vi "CBSControlling.vi"() -> ()   [LabVIEW 2017]
uses:
  classes/DataHandlerMYiTOPS.lvclass
panel:
  in  "Monitoring":T1 {"Meter" scale=0.0..20.0}
  out "appended array":string[](array[string])
  out "element":string
  out "Control-Matrix-Overview 2":i32(listbox)=-1
  in  "Controlling":T2
  in  "Cyber-physical Objects":i32(listbox)
  in  "Stop":bool
  out "Control-Matrix-Overview":i32(listbox)=-1
  # "Hard Key:"
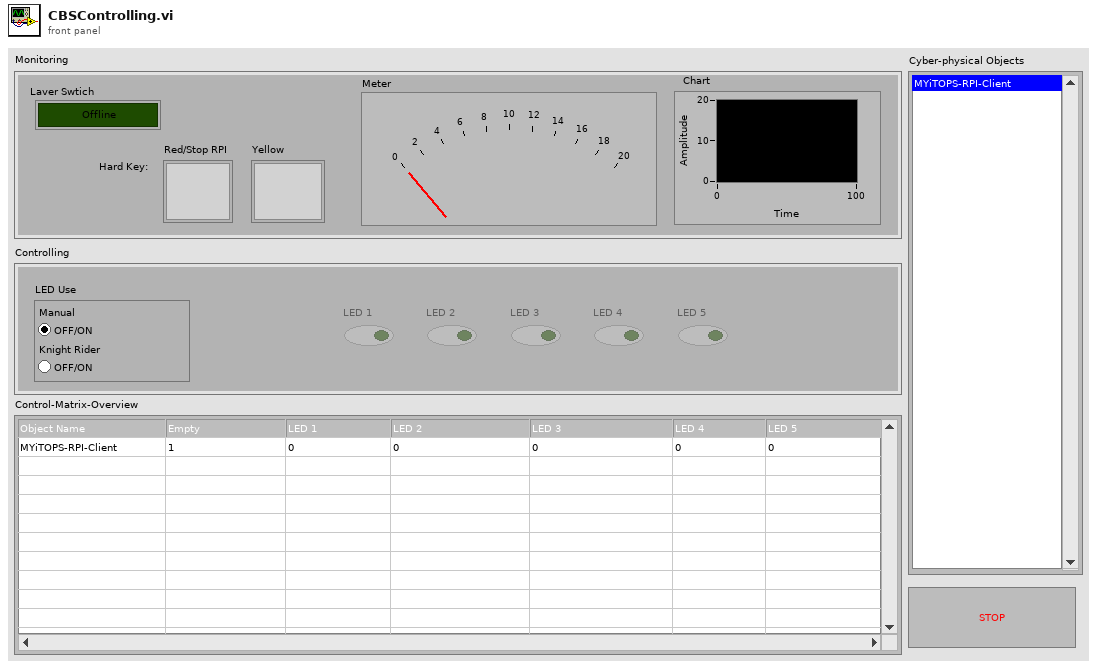
[diagram p1: front panel]
types:
  T1 = cluster{"Meter":i8, "Chart":dbl, "Yellow":bool, "Red/Stop RPI":bool, "Laver Swtich":bool}
  T2 = cluster{"LED 1":bool, "LED 5":bool, "LED 2":bool, "LED 3":bool, "LED 4":bool, "LED Use":enum32{"Manual", "Knight Rider"}}
  T3 = enum8{"Enabled", "Disabled", "Disabled and Grayed Out"}
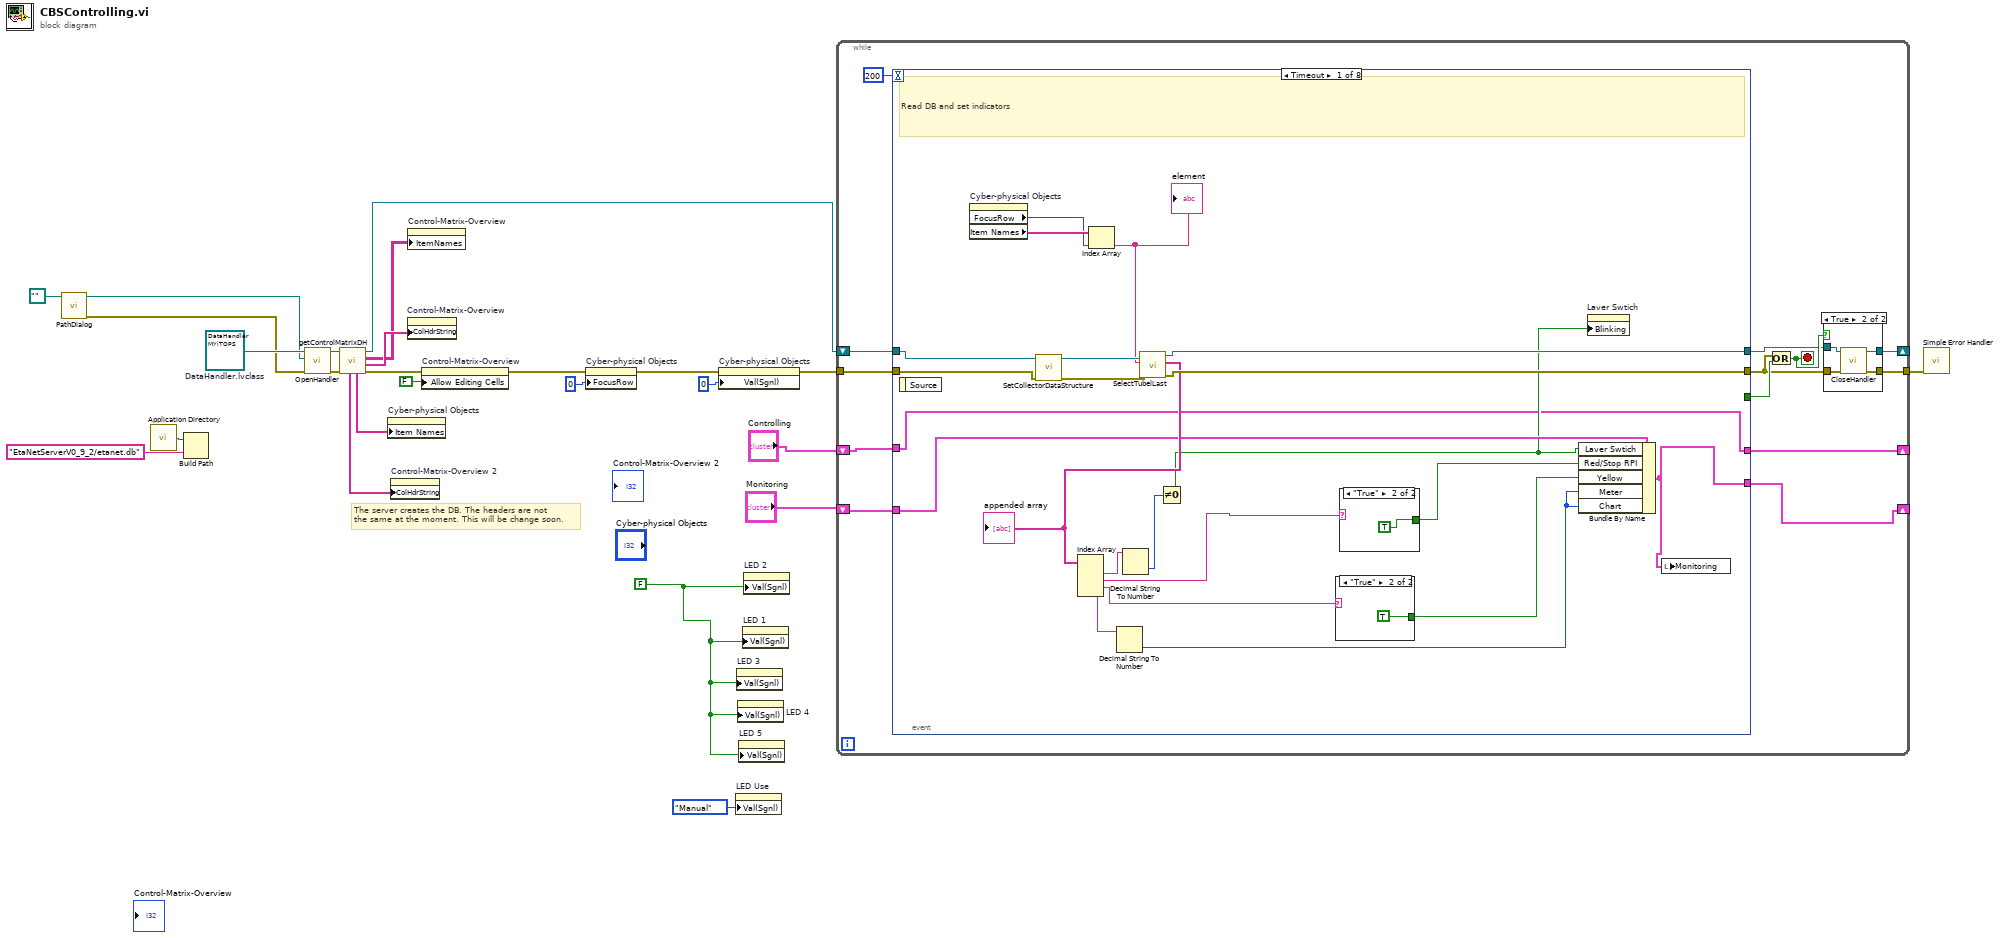
[diagram p0: block diagram]
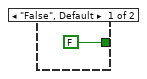
[diagram p3: hidden frame]
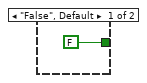
[diagram p4: hidden frame]
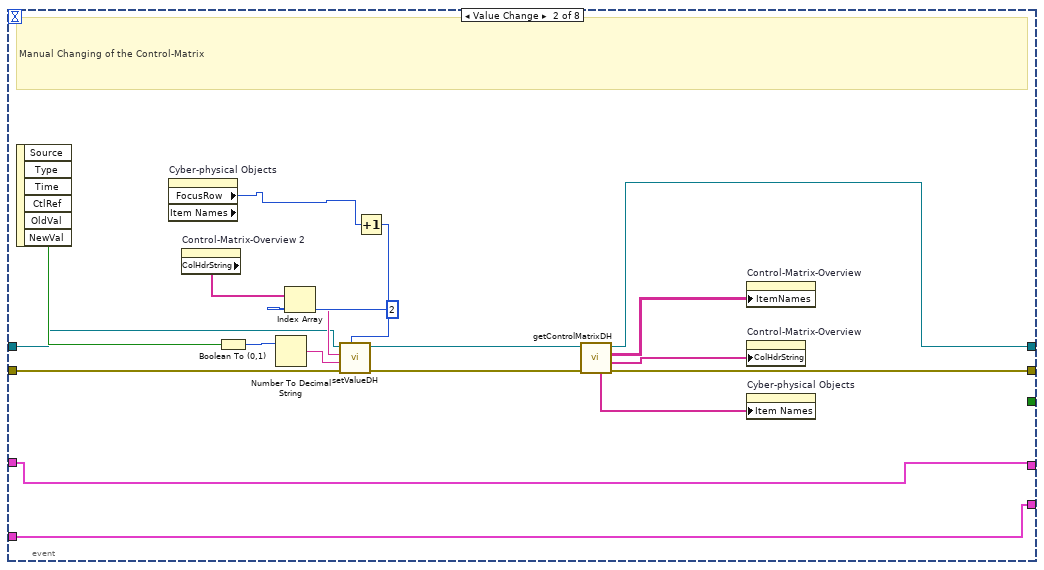
[diagram p5: hidden frame]
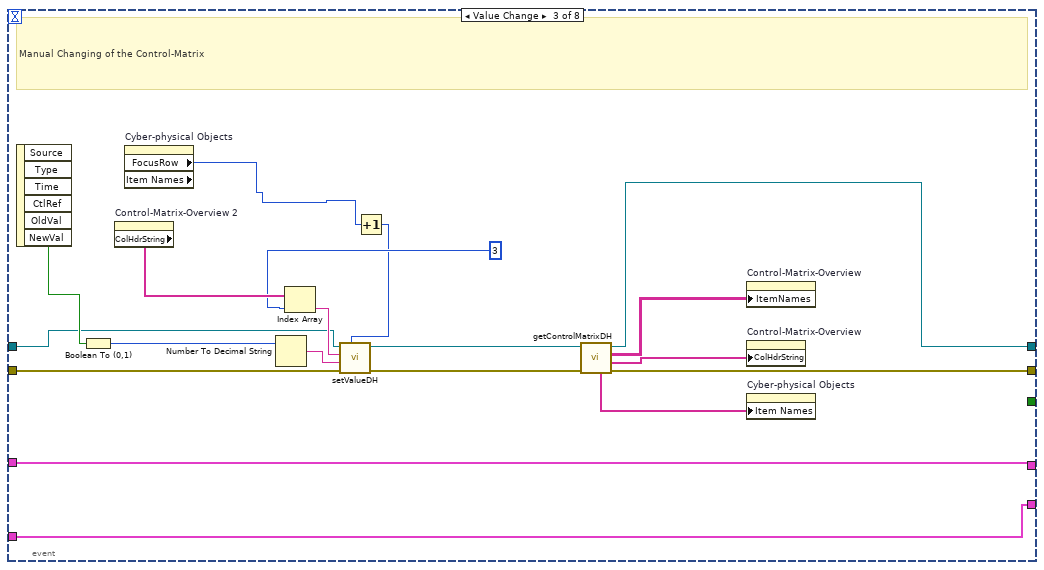
[diagram p6: hidden frame]
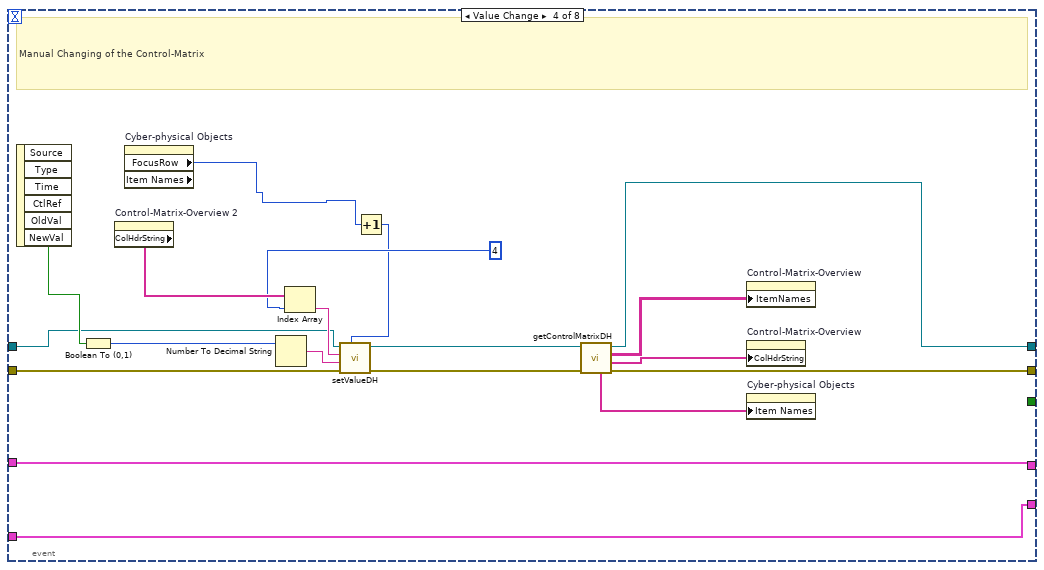
[diagram p7: hidden frame]
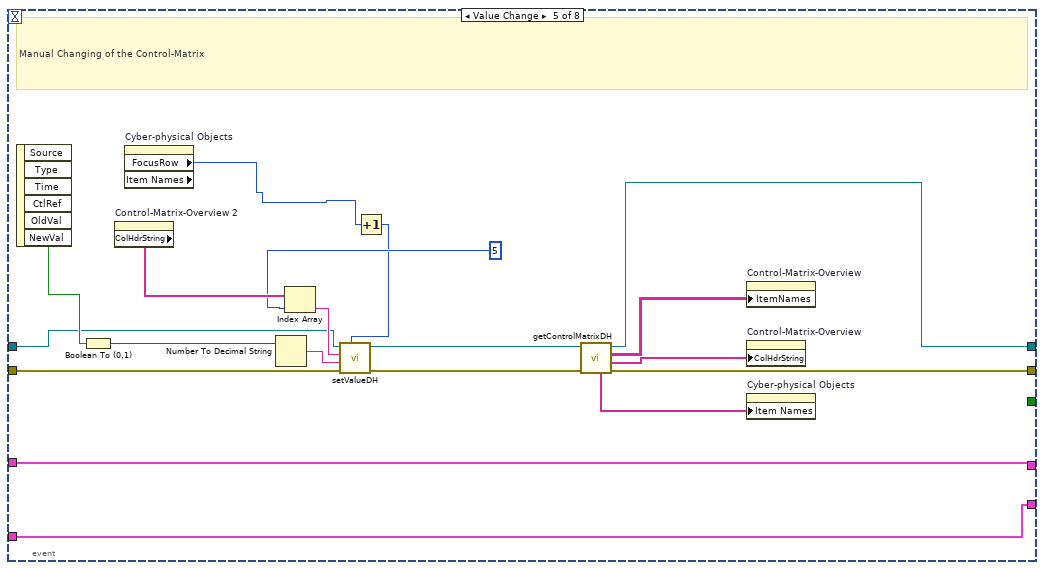
[diagram p8: hidden frame]
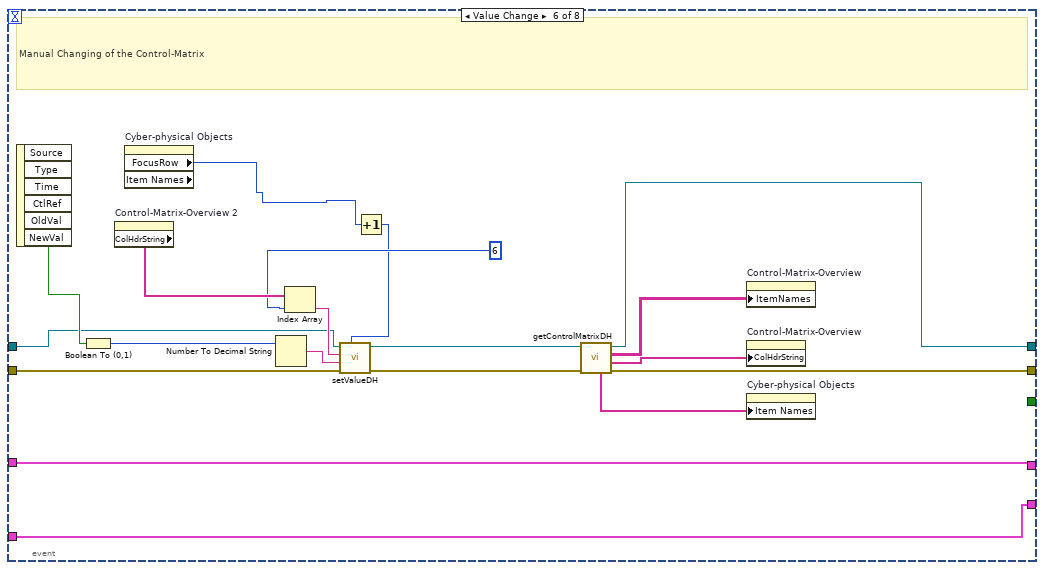
[diagram p9: hidden frame]
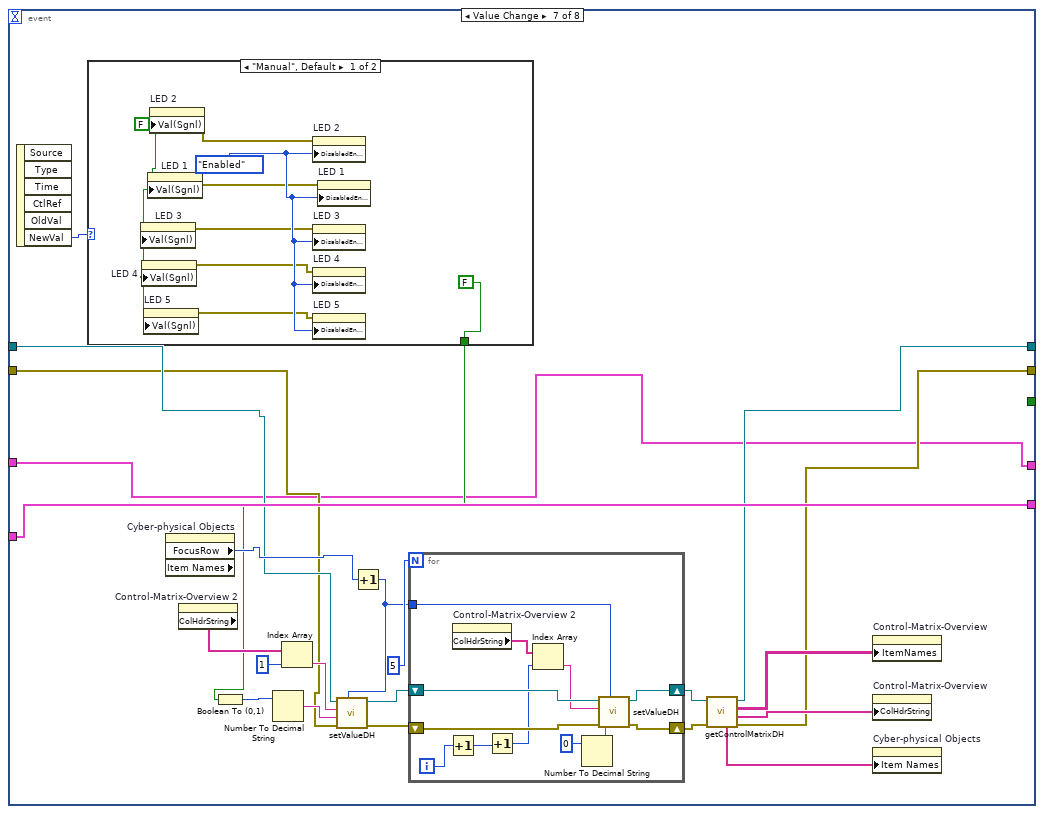
[diagram p10: hidden frame]
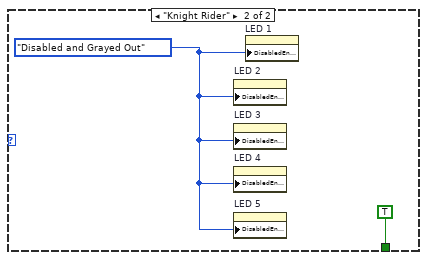
[diagram p11: hidden frame]
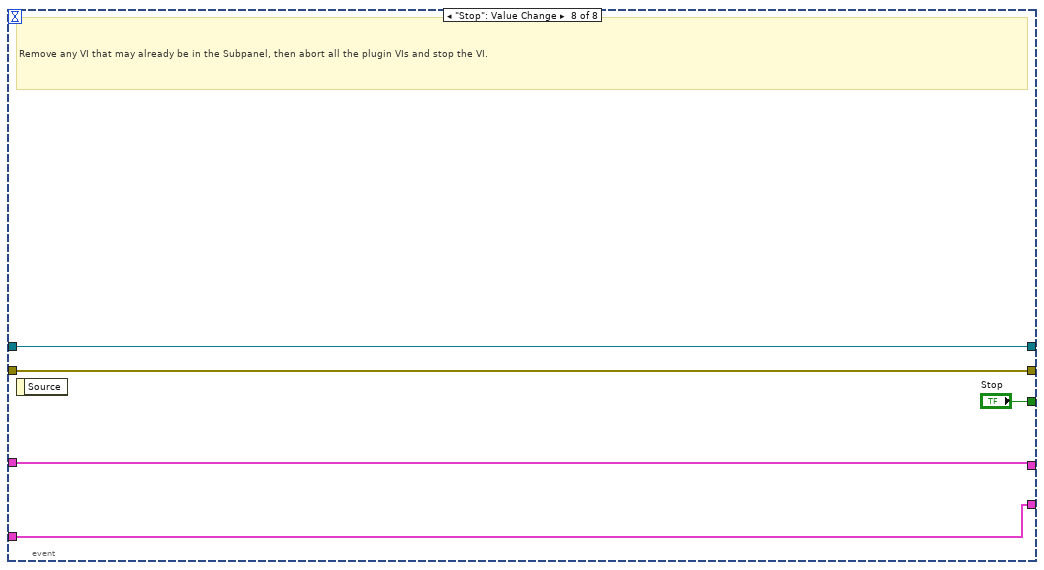
[diagram p12: hidden frame]
diagram:
  w4 = FALSE ("Value")
  w20 = refnum<class "DataHandlerMYiTOPS.lvclass"> refnum  # DataHandler.lvclass
  # "The server creates the DB. The headers are not \nthe same at the moment. This will be change soon."
  n1 = call "PathDialog.vi"("Path to Data Base in"=path "" ("Path to Data Base")) -> ("error out"=w2:errorcluster, "Path to Data Base out"=w6:path)  [unwired: 9 in]
  n2 = call <vilib>:"Application Directory.vi"() -> ("Application Directory"=w21:path)
  n3 = Build Path(base path=w21, name or relative path="EtaNetServerV0_9_2/etanet.db" ("Name oder relativer Pfad")) -> ()  [unwired: 1 out]
  n4 = call-dynamic "OpenHandler.vi"("error in (no error)"=w2, "path to db monitoring"=w6, "DataHandling in"=w20) -> ("error out"=w18:errorcluster, "DataHandling out"=w17:refnum<class "DataHandlerMYiTOPS.lvclass">)  [unwired: 7 in]
  n5 = call-dynamic "getControlMatrixDH.vi"("error in (no error)"=w18, "DataHandler in"=w17) -> ("error out"=w15:errorcluster, "List of ColHads"=w14:string[], "Array"=w9:string[][], "DataHandler out"=w10:refnum<class "DataHandlerMYiTOPS.lvclass">, "Field Elements"=w16:string[], "List of ColHads 2"=w8:string[])  [unwired: 4 in]
  n6 = property on="Cyber-physical Objects" class="LstBox (strict)"("Item Names"=w16) -> ()  [unwired: 2 in, 2 out]
  n7 = property on="Control-Matrix-Overview 2" class="MCListbox (strict)"("ColHdrString"=w8) -> ()  [unwired: 2 in, 2 out]
  n8 = property on="Control-Matrix-Overview" class="MCListbox (strict)"("ColHdrString"=w14) -> ()  [unwired: 2 in, 2 out]
  n9 = property on="Control-Matrix-Overview" class="MCListbox (strict)"("ItemNames"=w9) -> ()  [unwired: 2 in, 2 out]
  n10 = property on="Control-Matrix-Overview" class="MCListbox (strict)"(error in=w15, "Allow Editing Cells"=FALSE) -> (error out=w11:errorcluster)  [unwired: 1 in, 1 out]
  n11 = property on="Cyber-physical Objects" class="LstBox (strict)"(error in=w11, "FocusRow"=0 ("Focus Row")) -> (error out=w12:errorcluster)  [unwired: 1 in, 1 out]
  n12 = property on="Cyber-physical Objects" class="ListBox (strict)"(error in=w12, "Val(Sgnl)"=u16 0 ("Value (Signaling)")) -> (error out=w25:errorcluster)  [unwired: 1 in, 1 out]
  n13 = property on="LED Use" class="RadioBtnsControl (strict)"("Val(Sgnl)"=enum32{"Manual", "Knight Rider"}."Manual" ("Value (Signaling)")) -> ()  [unwired: 2 in, 2 out]
  n14 = property on="LED 3" class="Bool (strict)"("Val(Sgnl)"=w4) -> ()  [unwired: 2 in, 2 out]
  n15 = property on="LED 4" class="Bool (strict)"("Val(Sgnl)"=w4) -> ()  [unwired: 2 in, 2 out]
  n16 = property on="LED 5" class="Bool (strict)"("Val(Sgnl)"=w4) -> ()  [unwired: 2 in, 2 out]
  n17 = property on="LED 1" class="Bool (strict)"("Val(Sgnl)"=w4) -> ()  [unwired: 2 in, 2 out]
  n18 = property on="LED 2" class="Bool (strict)"("Val(Sgnl)"=w4) -> ()  [unwired: 2 in, 2 out]
  n19 = while {
    tunnel: w25 -> [w37]
    tunnel: [w32] -> w23
    shift-right: [w30] -> _
    shift-left: w10 -> [w35]
    shift-right: [w26] -> _
    shift-left: "Controlling" -> [w29]
    shift-right: [w27] -> _
    shift-left: "Monitoring" -> [w28]
    stop <- w34 stop-if-true
    n20 = event shown="[0] Timeout" {
      selector: _ -> [_ _ _ _ _ _ _ _]
      dyn-events: _ -> [_ _ _ _ _ _ _ _]
      timeout: 200 -> [_ _ _ _ _ _ _ _]
      tunnel: [_ _ _ _ _ _ _ "Stop"] -> w38
      tunnel: [w59 w87 w104 w123 w142 w161 w173 w213] -> w33
      tunnel: w37 -> [w61 w89 w108 w127 w146 w165 w174 w213]
      tunnel: w35 -> [w64 w78 w95 w114 w133 w152 w176 w214]
      tunnel: [w62 w79 w96 w115 w134 w153 w175 w214] -> w31
      tunnel: w29 -> [w45 w75 w91 w110 w129 w148 w166 w212]
      tunnel: [w45 w75 w91 w110 w129 w148 w166 w212] -> w26
      tunnel: w28 -> [w49 w74 w90 w109 w128 w147 w187 w211]
      tunnel: [w48 w74 w90 w109 w128 w147 w187 w211] -> w27
      event Timeout {
        # "Read DB and set indicators"
        n21 = event-data() -> ()  [unwired: 1 in, 1 out]
        n22 = property on="Cyber-physical Objects" class="LstBox (strict)"() -> ("FocusRow"=w65:i32, "Item Names"=w66:string[])  [unwired: 2 in, 2 out]
        n23 = call-dynamic "SetCollectorDataStructure.vi"("error in (no error)"=w61, "DataHandler in"=w64) -> ("error out"=w60:errorcluster, "DataHandler out"=w63:refnum<class "DataHandlerMYiTOPS.lvclass">)  [unwired: 8 in]
        n24 = Index Array(array=w66, index=w65) -> (element=w58:string)
        "element" <- w58
        n25 = call-dynamic "SelectTubelLast.vi"("error in (no error)"=w60, "Unique Object Identifier"=w58, "DataHandler in"=w63) -> ("error out"=w59:errorcluster, "appended array"=w57:string[], "DataHandler out"=w62:refnum<class "DataHandlerMYiTOPS.lvclass">)  [unwired: 6 in]
        "appended array" <- w57
        n26 = Index Array(array=w57) -> (element #1=w56:string, element #2=w55:string, element #3=w54:string, element #4=w53:string)  [unwired: 4 in]
        n27 = Decimal String To Number(string=w53) -> (number=w52:i32)  [unwired: 2 in, 1 out]
        n28 = Decimal String To Number(string=w56) -> (number=w47:i32)  [unwired: 2 in, 1 out]
        n29 = Not Equal To 0?(x=w47) -> (x != 0?=w46:bool)
        n30 = case shown="\"True\"" w54 {
          tunnel: [FALSE TRUE] -> w51
          frame "False", Default {
          }
          frame "True" {
          }
        }
        n31 = case shown="\"True\"" w55 {
          tunnel: [FALSE TRUE] -> w50
          frame "False", Default {
          }
          frame "True" {
          }
        }
        n32 = Bundle By Name(cluster=w49, "Laver Swtich"=w46, "Red/Stop RPI"=w50, "Yellow"=w51, "Meter"=w52, "Chart"=w52) -> (w48:T1)
        n33 = property on="Laver Swtich" class="Bool (strict)"("Blinking"=w46) -> ()  [unwired: 2 in, 2 out]
        n34 = local write "Monitoring"(w48) -> ()
      }
      event "Controlling.LED 1": Value Change {
        # "Manual Changing of the Control-Matrix"
        n35 = event-data() -> ("NewVal"=w82:bool)  [unwired: 1 in, 5 out]
        n36 = property on="Cyber-physical Objects" class="LstBox (strict)" props=["FocusRow", "Item Names"]() -> ("FocusRow"=w77:i32)  [unwired: 2 in, 3 out]
        n37 = property on="Control-Matrix-Overview 2" class="MCListbox (strict)"() -> ("ColHdrString"=w85:string[])  [unwired: 2 in, 2 out]
        n38 = Boolean To (0,1)(Boolean=w82) -> (0, 1=w81:i16)
        n39 = Number To Decimal String(number=w81) -> (decimal integer string=w86:string)  [unwired: 1 in]
        n40 = Index Array(array=w85, index=2) -> (element=w83:string)
        n41 = Increment(x=w77) -> (x+1=w76:i32)
        n42 = call-dynamic "setValueDH.vi"("Focus"=w76, "error in (no error)"=w89, "Value"=w86, "ItemName"=w83, "DataHandler in"=w78) -> ("error out"=w88:errorcluster, "DataHandler out"=w80:refnum<class "DataHandlerMYiTOPS.lvclass">)  [unwired: 5 in]
        n43 = call-dynamic "getControlMatrixDH.vi"("error in (no error)"=w88, "DataHandler in"=w80) -> ("error out"=w87:errorcluster, "List of ColHads"=w72:string[], "Array"=w71:string[][], "DataHandler out"=w79:refnum<class "DataHandlerMYiTOPS.lvclass">, "Field Elements"=w73:string[])  [unwired: 4 in, 1 out]
        n44 = property on="Control-Matrix-Overview" class="MCListbox (strict)"("ItemNames"=w71) -> ()  [unwired: 2 in, 2 out]
        n45 = property on="Control-Matrix-Overview" class="MCListbox (strict)"("ColHdrString"=w72) -> ()  [unwired: 2 in, 2 out]
        n46 = property on="Cyber-physical Objects" class="LstBox (strict)"("Item Names"=w73) -> ()  [unwired: 2 in, 2 out]
      }
      event "Controlling.LED 2": Value Change {
        # "Manual Changing of the Control-Matrix"
        n47 = event-data() -> ("NewVal"=w99:bool)  [unwired: 1 in, 5 out]
        n48 = Boolean To (0,1)(Boolean=w99) -> (0, 1=w98:i16)
        n49 = property on="Control-Matrix-Overview 2" class="MCListbox (strict)"() -> ("ColHdrString"=w102:string[])  [unwired: 2 in, 2 out]
        n50 = property on="Cyber-physical Objects" class="LstBox (strict)" props=["FocusRow", "Item Names"]() -> ("FocusRow"=w93:i32)  [unwired: 2 in, 3 out]
        n51 = Number To Decimal String(number=w98) -> (decimal integer string=w103:string)  [unwired: 1 in]
        n52 = Index Array(array=w102, index=3) -> (element=w100:string)
        n53 = Increment(x=w93) -> (x+1=w92:i32)
        n54 = call-dynamic "setValueDH.vi"("Focus"=w92, "error in (no error)"=w108, "Value"=w103, "ItemName"=w100, "DataHandler in"=w95) -> ("error out"=w105:errorcluster, "DataHandler out"=w97:refnum<class "DataHandlerMYiTOPS.lvclass">)  [unwired: 5 in]
        n55 = call-dynamic "getControlMatrixDH.vi"("error in (no error)"=w105, "DataHandler in"=w97) -> ("error out"=w104:errorcluster, "List of ColHads"=w106:string[], "Array"=w94:string[][], "DataHandler out"=w96:refnum<class "DataHandlerMYiTOPS.lvclass">, "Field Elements"=w107:string[])  [unwired: 4 in, 1 out]
        n56 = property on="Control-Matrix-Overview" class="MCListbox (strict)"("ItemNames"=w94) -> ()  [unwired: 2 in, 2 out]
        n57 = property on="Control-Matrix-Overview" class="MCListbox (strict)"("ColHdrString"=w106) -> ()  [unwired: 2 in, 2 out]
        n58 = property on="Cyber-physical Objects" class="LstBox (strict)"("Item Names"=w107) -> ()  [unwired: 2 in, 2 out]
      }
      event "Controlling.LED 3": Value Change {
        # "Manual Changing of the Control-Matrix"
        n59 = event-data() -> ("NewVal"=w118:bool)  [unwired: 1 in, 5 out]
        n60 = Boolean To (0,1)(Boolean=w118) -> (0, 1=w117:i16)
        n61 = property on="Control-Matrix-Overview 2" class="MCListbox (strict)"() -> ("ColHdrString"=w121:string[])  [unwired: 2 in, 2 out]
        n62 = property on="Cyber-physical Objects" class="LstBox (strict)" props=["FocusRow", "Item Names"]() -> ("FocusRow"=w112:i32)  [unwired: 2 in, 3 out]
        n63 = Number To Decimal String(number=w117) -> (decimal integer string=w122:string)  [unwired: 1 in]
        n64 = Index Array(array=w121, index=4) -> (element=w119:string)
        n65 = Increment(x=w112) -> (x+1=w111:i32)
        n66 = call-dynamic "setValueDH.vi"("Focus"=w111, "error in (no error)"=w127, "Value"=w122, "ItemName"=w119, "DataHandler in"=w114) -> ("error out"=w124:errorcluster, "DataHandler out"=w116:refnum<class "DataHandlerMYiTOPS.lvclass">)  [unwired: 5 in]
        n67 = call-dynamic "getControlMatrixDH.vi"("error in (no error)"=w124, "DataHandler in"=w116) -> ("error out"=w123:errorcluster, "List of ColHads"=w125:string[], "Array"=w113:string[][], "DataHandler out"=w115:refnum<class "DataHandlerMYiTOPS.lvclass">, "Field Elements"=w126:string[])  [unwired: 4 in, 1 out]
        n68 = property on="Control-Matrix-Overview" class="MCListbox (strict)"("ItemNames"=w113) -> ()  [unwired: 2 in, 2 out]
        n69 = property on="Control-Matrix-Overview" class="MCListbox (strict)"("ColHdrString"=w125) -> ()  [unwired: 2 in, 2 out]
        n70 = property on="Cyber-physical Objects" class="LstBox (strict)"("Item Names"=w126) -> ()  [unwired: 2 in, 2 out]
      }
      event "Controlling.LED 4": Value Change {
        # "Manual Changing of the Control-Matrix"
        n71 = event-data() -> ("NewVal"=w137:bool)  [unwired: 1 in, 5 out]
        n72 = Boolean To (0,1)(Boolean=w137) -> (0, 1=w136:i16)
        n73 = property on="Control-Matrix-Overview 2" class="MCListbox (strict)"() -> ("ColHdrString"=w140:string[])  [unwired: 2 in, 2 out]
        n74 = property on="Cyber-physical Objects" class="LstBox (strict)" props=["FocusRow", "Item Names"]() -> ("FocusRow"=w131:i32)  [unwired: 2 in, 3 out]
        n75 = Number To Decimal String(number=w136) -> (decimal integer string=w141:string)  [unwired: 1 in]
        n76 = Index Array(array=w140, index=5) -> (element=w138:string)
        n77 = Increment(x=w131) -> (x+1=w130:i32)
        n78 = call-dynamic "setValueDH.vi"("Focus"=w130, "error in (no error)"=w146, "Value"=w141, "ItemName"=w138, "DataHandler in"=w133) -> ("error out"=w143:errorcluster, "DataHandler out"=w135:refnum<class "DataHandlerMYiTOPS.lvclass">)  [unwired: 5 in]
        n79 = call-dynamic "getControlMatrixDH.vi"("error in (no error)"=w143, "DataHandler in"=w135) -> ("error out"=w142:errorcluster, "List of ColHads"=w144:string[], "Array"=w132:string[][], "DataHandler out"=w134:refnum<class "DataHandlerMYiTOPS.lvclass">, "Field Elements"=w145:string[])  [unwired: 4 in, 1 out]
        n80 = property on="Control-Matrix-Overview" class="MCListbox (strict)"("ItemNames"=w132) -> ()  [unwired: 2 in, 2 out]
        n81 = property on="Control-Matrix-Overview" class="MCListbox (strict)"("ColHdrString"=w144) -> ()  [unwired: 2 in, 2 out]
        n82 = property on="Cyber-physical Objects" class="LstBox (strict)"("Item Names"=w145) -> ()  [unwired: 2 in, 2 out]
      }
      event "Controlling.LED 5": Value Change {
        # "Manual Changing of the Control-Matrix"
        n83 = event-data() -> ("NewVal"=w156:bool)  [unwired: 1 in, 5 out]
        n84 = Boolean To (0,1)(Boolean=w156) -> (0, 1=w155:i16)
        n85 = property on="Control-Matrix-Overview 2" class="MCListbox (strict)"() -> ("ColHdrString"=w159:string[])  [unwired: 2 in, 2 out]
        n86 = property on="Cyber-physical Objects" class="LstBox (strict)" props=["FocusRow", "Item Names"]() -> ("FocusRow"=w150:i32)  [unwired: 2 in, 3 out]
        n87 = Number To Decimal String(number=w155) -> (decimal integer string=w160:string)  [unwired: 1 in]
        n88 = Index Array(array=w159, index=6) -> (element=w157:string)
        n89 = Increment(x=w150) -> (x+1=w149:i32)
        n90 = call-dynamic "setValueDH.vi"("Focus"=w149, "error in (no error)"=w165, "Value"=w160, "ItemName"=w157, "DataHandler in"=w152) -> ("error out"=w162:errorcluster, "DataHandler out"=w154:refnum<class "DataHandlerMYiTOPS.lvclass">)  [unwired: 5 in]
        n91 = call-dynamic "getControlMatrixDH.vi"("error in (no error)"=w162, "DataHandler in"=w154) -> ("error out"=w161:errorcluster, "List of ColHads"=w163:string[], "Array"=w151:string[][], "DataHandler out"=w153:refnum<class "DataHandlerMYiTOPS.lvclass">, "Field Elements"=w164:string[])  [unwired: 4 in, 1 out]
        n92 = property on="Control-Matrix-Overview" class="MCListbox (strict)"("ItemNames"=w151) -> ()  [unwired: 2 in, 2 out]
        n93 = property on="Control-Matrix-Overview" class="MCListbox (strict)"("ColHdrString"=w163) -> ()  [unwired: 2 in, 2 out]
        n94 = property on="Cyber-physical Objects" class="LstBox (strict)"("Item Names"=w164) -> ()  [unwired: 2 in, 2 out]
      }
      event "Controlling.LED Use": Value Change {
        n95 = event-data() -> ("NewVal"=w188:enum32{"Manual", "Knight Rider"})  [unwired: 1 in, 5 out]
        n96 = case shown="\"Manual\", Default" w188 {
          tunnel: [FALSE TRUE] -> w177
          frame "Manual", Default {
            w205 = FALSE ("Value")
            w208 = T3."Enabled" ("Disabled")
            n97 = property on="LED 3" class="Bool (strict)"("Val(Sgnl)"=w205) -> (error out=w203:errorcluster)  [unwired: 2 in, 1 out]
            n98 = property on="LED 4" class="Bool (strict)"("Val(Sgnl)"=w205) -> (error out=w202:errorcluster)  [unwired: 2 in, 1 out]
            n99 = property on="LED 5" class="Bool (strict)"("Val(Sgnl)"=w205) -> (error out=w201:errorcluster)  [unwired: 2 in, 1 out]
            n100 = property on="LED 1" class="Bool (strict)"("Val(Sgnl)"=w205) -> (error out=w204:errorcluster)  [unwired: 2 in, 1 out]
            n101 = property on="LED 2" class="Bool (strict)"("Val(Sgnl)"=w205) -> (error out=w206:errorcluster)  [unwired: 2 in, 1 out]
            n102 = property on="LED 2" class="Bool (strict)"(error in=w206, "DisabledEnum"=w208) -> ()  [unwired: 1 in, 2 out]
            n103 = property on="LED 3" class="Bool (strict)"(error in=w203, "DisabledEnum"=w208) -> ()  [unwired: 1 in, 2 out]
            n104 = property on="LED 4" class="Bool (strict)"(error in=w202, "DisabledEnum"=w208) -> ()  [unwired: 1 in, 2 out]
            n105 = property on="LED 5" class="Bool (strict)"(error in=w201, "DisabledEnum"=w208) -> ()  [unwired: 1 in, 2 out]
            n106 = property on="LED 1" class="Bool (strict)"(error in=w204, "DisabledEnum"=w208) -> ()  [unwired: 1 in, 2 out]
          }
          frame "Knight Rider" {
            w210 = T3."Disabled and Grayed Out" ("Disabled")
            n107 = property on="LED 2" class="Bool (strict)"("DisabledEnum"=w210) -> ()  [unwired: 2 in, 2 out]
            n108 = property on="LED 3" class="Bool (strict)"("DisabledEnum"=w210) -> ()  [unwired: 2 in, 2 out]
            n109 = property on="LED 4" class="Bool (strict)"("DisabledEnum"=w210) -> ()  [unwired: 2 in, 2 out]
            n110 = property on="LED 5" class="Bool (strict)"("DisabledEnum"=w210) -> ()  [unwired: 2 in, 2 out]
            n111 = property on="LED 1" class="Bool (strict)"("DisabledEnum"=w210) -> ()  [unwired: 2 in, 2 out]
          }
        }
        n112 = property on="Cyber-physical Objects" class="LstBox (strict)" props=["FocusRow", "Item Names"]() -> ("FocusRow"=w182:i32)  [unwired: 2 in, 3 out]
        n113 = property on="Control-Matrix-Overview 2" class="MCListbox (strict)"() -> ("ColHdrString"=w185:string[])  [unwired: 2 in, 2 out]
        n114 = Boolean To (0,1)(Boolean=w177) -> (0, 1=w183:i16)
        n115 = Number To Decimal String(number=w183) -> (decimal integer string=w186:string)  [unwired: 1 in]
        n116 = Index Array(array=w185, index=1) -> (element=w184:string)
        n117 = Increment(x=w182) -> (x+1=w167:i32)
        n118 = call-dynamic "setValueDH.vi"("Focus"=w167, "error in (no error)"=w174, "Value"=w186, "ItemName"=w184, "DataHandler in"=w176) -> ("error out"=w172:errorcluster, "DataHandler out"=w170:refnum<class "DataHandlerMYiTOPS.lvclass">)  [unwired: 5 in]
        n119 = for {
          N: 5 -> [_]
          shift-right: [w199] -> w171
          shift-left: w172 -> [w200]
          shift-right: [w197] -> w169
          shift-left: w170 -> [w198]
          tunnel: w167 -> [w190]
          i -> [w195]
          n120 = Increment(x=w195) -> (x+1=w194:i32)
          n121 = property on="Control-Matrix-Overview 2" class="MCListbox (strict)"() -> ("ColHdrString"=w193:string[])  [unwired: 2 in, 2 out]
          n122 = Increment(x=w194) -> (x+1=w192:i32)
          n123 = Index Array(array=w193, index=w192) -> (element=w191:string)
          n124 = Number To Decimal String(number=0) -> (decimal integer string=w196:string)  [unwired: 1 in]
          n125 = call-dynamic "setValueDH.vi"("Focus"=w190, "error in (no error)"=w200, "Value"=w196, "ItemName"=w191, "DataHandler in"=w198) -> ("error out"=w199:errorcluster, "DataHandler out"=w197:refnum<class "DataHandlerMYiTOPS.lvclass">)  [unwired: 5 in]
        }
        n126 = call-dynamic "getControlMatrixDH.vi"("error in (no error)"=w171, "DataHandler in"=w169) -> ("error out"=w173:errorcluster, "List of ColHads"=w180:string[], "Array"=w179:string[][], "DataHandler out"=w175:refnum<class "DataHandlerMYiTOPS.lvclass">, "Field Elements"=w181:string[])  [unwired: 4 in, 1 out]
        n127 = property on="Control-Matrix-Overview" class="MCListbox (strict)"("ItemNames"=w179) -> ()  [unwired: 2 in, 2 out]
        n128 = property on="Control-Matrix-Overview" class="MCListbox (strict)"("ColHdrString"=w180) -> ()  [unwired: 2 in, 2 out]
        n129 = property on="Cyber-physical Objects" class="LstBox (strict)"("Item Names"=w181) -> ()  [unwired: 2 in, 2 out]
      }
      event "Stop": Value Change {
        # "Remove any VI that may already be in the Subpanel, then abort all the plugin VIs and stop the VI."
        n130 = event-data() -> ()  [unwired: 1 in, 1 out]
      }
    }
    n131 = Or(x=w33, y=w38) -> (x .or. y?=w34:bool)
    n132 = case shown="True" w34 {
      tunnel: w33 -> [w40 w43]
      tunnel: [w40 w44] -> w32
      tunnel: w31 -> [w39 w42]
      tunnel: [w39 w41] -> w30
      frame False {
      }
      frame True {
        n133 = call-dynamic "CloseHandler.vi"("error in (no error)"=w43, "DataHandling in"=w42) -> ("error out"=w44:errorcluster, "DataHandling out"=w41:refnum<class "DataHandlerMYiTOPS.lvclass">)  [unwired: 8 in]
      }
    }
  }
  n134 = call <vilib>:"Simple Error Handler.vi"("error in (no error)"=w23) -> ()  [unwired: 4 in, 5 out]
